vi "Basic Example.vi"() -> ()   [LabVIEW 2019]
uses:
  <vilib>/addons/VeriStand Custom Device Scripting APIs/Instrument Addon/Libraries Directory/Protocols.lvlibp/TCP/TCP Settings.ctl
  <vilib>/addons/VeriStand Custom Device Scripting APIs/Instrument Addon/API/TypeDefs/Command Settings.ctl
  <vilib>/NI VeriStand/Custom Device API/Custom Device Item Ref.ctl
  <vilib>/addons/VeriStand Custom Device Scripting APIs/Instrument Addon/API/TypeDefs/Padding.ctl
  <vilib>/addons/VeriStand Custom Device Scripting APIs/Instrument Addon/API/TypeDefs/Wait Response Settings.ctl
  <vilib>/addons/VeriStand Custom Device Scripting APIs/Instrument Addon/API/TypeDefs/Linked Channel.ctl
  <vilib>/addons/VeriStand Custom Device Scripting APIs/Instrument Addon/API/Custom Device/TCP Factory.vi
  <vilib>/addons/VeriStand Custom Device Scripting APIs/Instrument Addon/API/Messages/Create Message - Trigger Only.vi
  <vilib>/addons/VeriStand Custom Device Scripting APIs/Instrument Addon/API/Messages/Configure Response - Wait (sec).vi
  <vilib>/addons/VeriStand Custom Device Scripting APIs/Instrument Addon/API/Instrument Addon Scripting API.lvlib
  <vilib>/addons/VeriStand Custom Device Scripting APIs/Instrument Addon/Libraries Directory/Protocols.lvlibp/TCP/TCP.lvclass
  <vilib>/NI VeriStand/Custom Device API/Custom Device API.lvlib
panel:
  in  "Exported Configuration File":path=path "Exported Configuration.dat"
  in  "Output System Definition File":path=path "System Definition Files/Basic Example Output.nivssdf"
  in  "Input System Definition File":path=path "System Definition Files/Base.nivssdf"
  # "Overview: Creates and configures an Instrument Addon Custom Device with a single message, both Command and Response, and exports the configuration to a file on disk.\n\nThe VI executes the following steps:\n1. Creates a new TCP Protocol object and uses the protocol as an input for a new Instrument Addon Custom Device.\n2. Updates the name of the add-on.\n3. Creates a message section and a new message.\n4. Adds and configures the Command and Response sections.\n5. Export configuration file to disk at the specified location.\n6. Save System Definition file at the specification location.\n\nNote: The settings input for the Configure Response uses a known value, 42, as the channel refnum for the linked channel. This channel is composed of a variable name and a channel refnum.\n\nInstructions:\n1. Browse to the system definition file to be used as input.\n2. Browse to a path to save the system definition file as output. This may be the same as the input file.\n3. Browse to a path to save the exported custom device configuration. This is used in other examples.\n4. Run the VI and verify its results."
  # "System Definition Files"
  # "Configuration Files"
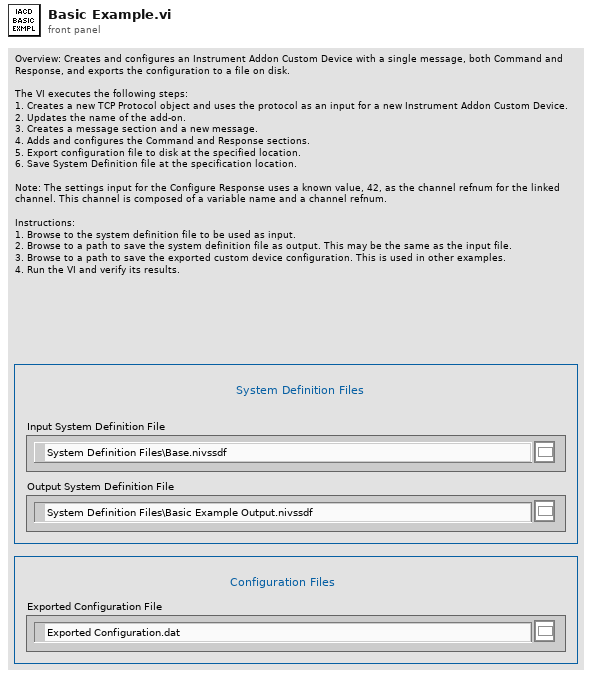
[diagram p1: front panel]
types:
  T1 = typedef "Instrument Addon Scripting API.lvlib/Wait Response Settings.ctl" = cluster{"Response Format":string, "Linked Channels":T2[], "Wait value (sec)":dbl, "Use Wait Channel":bool, "Channel Refnum":T3}
  T2 = typedef "Instrument Addon Scripting API.lvlib/Linked Channel.ctl" = cluster{"Variable Name":string, "Channel Refnum":T3}
  T3 = typedef "Custom Device API.lvlib/Custom Device Item Ref.ctl" = u64
  T4 = typedef "Instrument Addon Scripting API.lvlib/Command Settings.ctl" = cluster{"Command Format":string, "Linked Channels":cluster{"Variable Name":string, "Channel Ref in":T3}[], "Use Padding?":bool, "Padding":T5}
  T5 = typedef "Instrument Addon Scripting API.lvlib/Padding.ctl" = cluster{"Pad Value":u8, "Length":u32}
  T6 = typedef "Protocols.lvlibp/TCP.lvclass/TCP Settings.ctl" = cluster{"IP Address":string, "Port":u16}
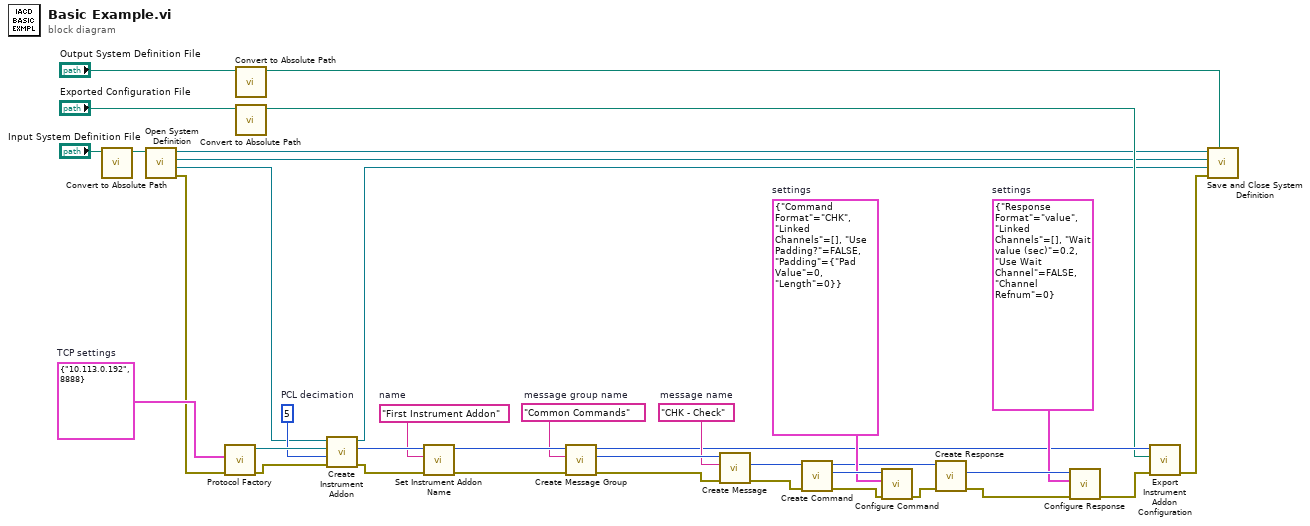
[diagram p0: block diagram]
diagram:
  w15 = T1 {"Response Format"="value", "Linked Channels"=[], "Wait value (sec)"=0.2, "Use Wait Channel"=FALSE, "Channel Refnum"=0}  # settings
  w21 = T4 {"Command Format"="CHK", "Linked Channels"=[], "Use Padding?"=FALSE, "Padding"={"Pad Value"=0, "Length"=0}}  # settings
  w26 = "CHK - Check"  # message name
  w28 = "Common Commands"  # message group name
  w32 = "First Instrument Addon"  # name
  w34 = u16 5  # PCL decimation
  w37 = T6 {"IP Address"="10.113.0.192", "Port"=8888}  # TCP settings
  n1 = call "Convert to Absolute Path.vi"("System Definition File"="Input System Definition File") -> ("Absolute Path"=w10:path)  [unwired: 10 in]
  n2 = call "Open System Definition.vi"("System Definition File"=w10) -> ("error out"=w11:errorcluster, "Target Refnum"=w9:refnum<k24>, "Root Refnum"=w4:refnum<k24>, "System Definition Refnum"=w5:refnum<k24>)  [unwired: 7 in]
  n3 = call-poly <vilib>:"Protocol Factory.vi"("error in (no error)"=w11, "settings"=w37) -> ("error out"=w35:errorcluster, "protocol out"=w36:refnum<class "Protocol Parent.lvclass">)  [unwired: 8 in]
  n4 = call "Convert to Absolute Path.vi"("System Definition File"="Output System Definition File") -> ("Absolute Path"=w1:path)  [unwired: 10 in]
  n5 = call "Convert to Absolute Path.vi"("System Definition File"="Exported Configuration File") -> ("Absolute Path"=w6:path)  [unwired: 10 in]
  n6 = call <vilib>:"Create Instrument Addon.vi"("error in (no error)"=w35, "PCL decimation"=w34, "protocol in"=w36, "target in"=w9) -> ("error out"=w31:errorcluster, "instrument addon refnum"=w33:T3, "target out"=w3:refnum<k24>)  [unwired: 5 in]
  n7 = call <vilib>:"Set Instrument Addon Name.vi"("error in (no error)"=w31, "name"=w32, "instrument addon refnum in"=w33) -> ("error out"=w29:errorcluster, "instrument addon refnum out"=w30:T3)  [unwired: 7 in]
  n8 = call <vilib>:"Create Message Group.vi"("error in (no error)"=w29, "message group name"=w28, "instrument addon refnum in"=w30) -> ("error out"=w25:errorcluster, "message group refnum out"=w27:T3, "instrument addon refnum out"=w14:T3)  [unwired: 6 in]
  n9 = call-poly <vilib>:"Create Message.vi"("error in (no error)"=w25, "message name"=w26, "message group refnum in"=w27) -> ("error out"=w23:errorcluster, "message refnum out"=w24:T3)  [unwired: 6 in, 1 out]
  n10 = call <vilib>:"Create Command.vi"("error in"=w23, "message refnum In"=w24) -> ("error out"=w20:errorcluster, "command refnum"=w22:T3, "message refnum out"=w19:T3)  [unwired: 7 in]
  n11 = call <vilib>:"Configure Command.vi"("error in (no error)"=w20, "settings"=w21, "command refnum in"=w22) -> ("error out"=w18:errorcluster)  [unwired: 7 in, 1 out]
  n12 = call <vilib>:"Create Response.vi"("error in (no error)"=w18, "message refnum in"=w19) -> ("error out"=w16:errorcluster, "response refnum"=w17:T3)  [unwired: 7 in, 1 out]
  n13 = call-poly <vilib>:"Configure Response.vi"("error in (no error)"=w16, "settings"=w15, "reponse refnum in"=w17) -> ("error out"=w13:errorcluster)  [unwired: 7 in, 1 out]
  n14 = call <vilib>:"Export Instrument Addon Configuration.vi"("error in (no error)"=w13, "export file path"=w6, "instrument addon refnum in"=w14) -> ("error out"=w2:errorcluster)  [unwired: 7 in, 1 out]
  n15 = call "Save and Close System Definition.vi"("System Definition Path"=w1, "error in (no error)"=w2, "Target Refnum"=w3, "Root Refnum"=w4, "System Definition Refnum"=w5) -> ()  [unwired: 6 in, 1 out]
